vi "GetWhereIGetMyInformation .vi"(8 "error in (no error)":errorcluster caption="Fehler (Eingang, kein Fehler)", 11 "ApplicationInititialisation (Eingang)":refnum<class "ApplicationInititialisation.lvclass">) -> (0 "error out":errorcluster caption="Fehler (Ausgang)", 2 "WhereIGetMyInformation":string, 3 "ApplicationInititialisation (Ausgang)":refnum<class "ApplicationInititialisation.lvclass">)   [LabVIEW 2013, in "ApplicationInititialisation.lvclass"]
uses:
  ApplicationInititialisation.lvclass
  ApplicationInititialisation.lvclass/ApplicationInititialisation.ctl
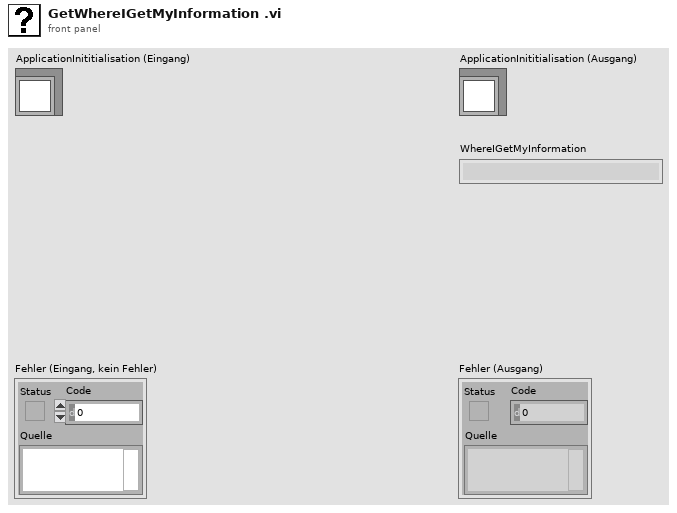
[diagram p1: front panel]
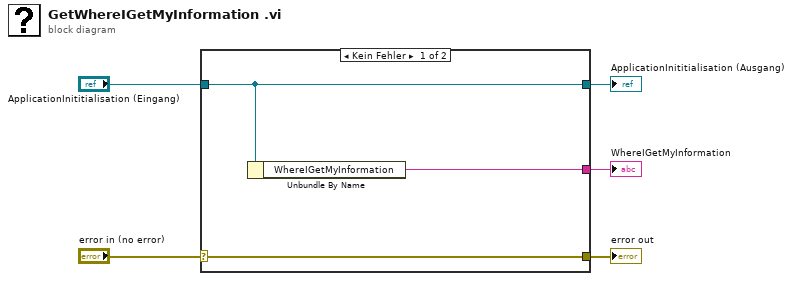
[diagram p0: block diagram]
diagram:
  n1 = case shown="Kein Fehler" "error in (no error)" {
    selector: "error in (no error)" -> [w8 w9]
    tunnel: [w8 w9] -> w4
    tunnel: [w7 w10] -> w2
    tunnel: "ApplicationInititialisation (Eingang)" -> [w7 w10]
    tunnel: [w6 _] -> w1
    frame No Error {
      n2 = Unbundle By Name(w7) -> ("WhereIGetMyInformation"=w6:string)
    }
    frame Error {
    }
  }
  "error out" <- w4
  "ApplicationInititialisation (Ausgang)" <- w2
  "WhereIGetMyInformation" <- w1
